vi "Manipulator Controller.vi"   [LabVIEW 2019]
uses:
  <vilib>/Rock Robotics/WPI/Joystick/WPI_JoystickDeviceEnum.ctl
  Manipulator Controller Gobal.vi
types:
  T1 = typedef "WPI_JoystickDeviceEnum.ctl" = enum16{"USB 0", "USB 1", "USB 2", "USB 3", "USB 4", "USB 5"}
  T2 = typedef "WPI_JoystickDevRef.ctl" = cluster{"Device":T1}
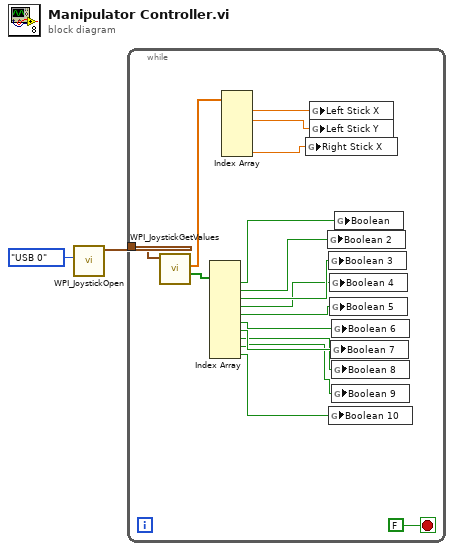
[diagram p0: block diagram]
diagram:
  n1 = call <vilib>:"WPI_JoystickOpen.vi"("JoystickDevice"=WPI_JoystickDeviceEnum."USB 0") -> ("JoystickDevRef"=w2:T2)  [unwired: 10 in]
  n2 = while {
    tunnel: w2 -> [w19]
    stop <- FALSE stop-if-true
    n3 = call <vilib>:"WPI_JoystickGetValues.vi"("JoystickDevRef"=w19) -> ("Buttons"=w18:bool[], "Axes"=w7:dbl[])  [unwired: 6 in, 3 out]
    n4 = Index Array(array=w18) -> (element #1=w17:bool, element #2=w16:bool, element #3=w15:bool, element #4=w14:bool, element #5=w13:bool, element #6=w12:bool, element #7=w11:bool, element #8=w10:bool, element #9=w9:bool, element #10=w8:bool)  [unwired: 10 in]
    n5 = Index Array(array=w7) -> (element #1=w6:dbl, element #2=w5:dbl, element #6=w4:dbl)  [unwired: 6 in, 3 out]
    n6 = global write "Manipulator Controller Gobal.vi" "Right Stick X"(w4) -> ()
    n7 = global write "Manipulator Controller Gobal.vi" "Left Stick X"(w6) -> ()
    n8 = global write "Manipulator Controller Gobal.vi" "Left Stick Y"(w5) -> ()
    n9 = global write "Manipulator Controller Gobal.vi" "Boolean 2"(w16) -> ()
    n10 = global write "Manipulator Controller Gobal.vi" "Boolean 3"(w15) -> ()
    n11 = global write "Manipulator Controller Gobal.vi" "Boolean 10"(w8) -> ()
    n12 = global write "Manipulator Controller Gobal.vi" "Boolean 4"(w14) -> ()
    n13 = global write "Manipulator Controller Gobal.vi" "Boolean 5"(w13) -> ()
    n14 = global write "Manipulator Controller Gobal.vi" "Boolean 7"(w11) -> ()
    n15 = global write "Manipulator Controller Gobal.vi" "Boolean 6"(w12) -> ()
    n16 = global write "Manipulator Controller Gobal.vi" "Boolean 8"(w10) -> ()
    n17 = global write "Manipulator Controller Gobal.vi" "Boolean 9"(w9) -> ()
    n18 = global write "Manipulator Controller Gobal.vi" "Boolean"(w17) -> ()
  }
